vi "To String.vi"(8 "error in (no error)":errorcluster, 11 "I32 in":refnum<class "I32.lvclass">) -> (0 "error out":errorcluster, 2 "String":string)   [LabVIEW 2020, in "Data.lvlib" / "I32.lvclass"]
doc: "Convert 'Generic Data in' to a string."
uses:
  I32.lvclass
  I32.lvclass/I32.ctl
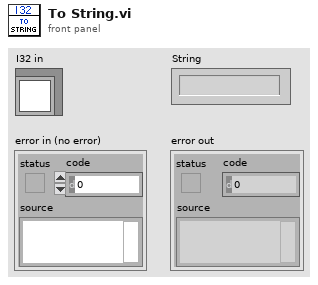
[diagram p1: front panel]
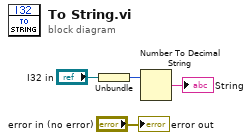
[diagram p0: block diagram]
diagram:
  n1 = Unbundle("I32 in") -> (w2:i32)
  n2 = Number To Decimal String(number=w2) -> (decimal integer string=→"String":string)  [unwired: 1 in]
  "error out" <- "error in (no error)"
